vi "CSGaussmeter.setactValue.vi"(0 "VisaCluster":T7, 7 "setValues":T6 {"Set_Rel"."Numeric" format="%#_4f"; "Set_upper"."Numeric" format="%#_4f"; "Set_lower"."Numeric" format="%#_4f"}, 11 "error in":errorcluster) -> (4 "VisaCluster 2":T7, 8 "setValues":T6 {"Set_Rel"."Numeric" format="%#_4f"; "Set_upper"."Numeric" format="%#_4f"; "Set_lower"."Numeric" format="%#_4f"}, 15 "error out":errorcluster)   [LabVIEW 2014, in "CSGaussmeter.lvlib"]
uses:
  CSGaussmeter.lvlib
  CSinstr.lib/FH_55/TypeDef/VisaCluster.ctl
  CSinstr.lib/FH_55/TypeDef/Unit.ctl
  CSinstr.lib/FH_55/TypeDef/Temp_Unit.ctl
  CSinstr.lib/FH_55/TypeDef/Max.ctl
  CSinstr.lib/FH_55/TypeDef/Range.ctl
  CSinstr.lib/FH_55/TypeDef/Unit2.ctl
  CSinstr.lib/FH_55/FH 55.lvlib
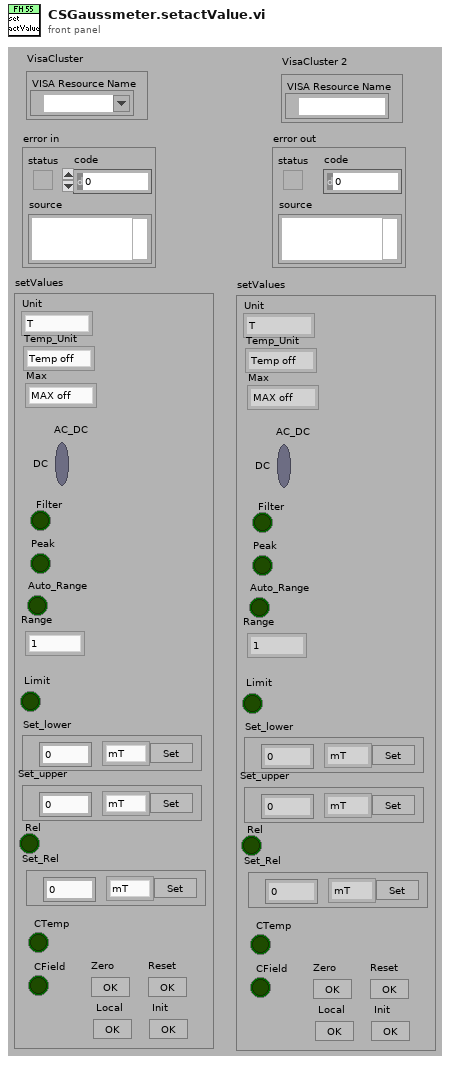
[diagram p1: front panel]
types:
  T1 = typedef "FH 55.lvlib/Unit.ctl" = enum16{"T", "G", "A/m"}
  T2 = typedef "FH 55.lvlib/Temp_Unit.ctl" = enum16{"Temp off", "Celsius", "Fahrenheit"}
  T3 = typedef "FH 55.lvlib/Max.ctl" = enum16{"MAX off", "Show MAX", "MAX/MIN"}
  T4 = typedef "FH 55.lvlib/Range.ctl" = enum16{"1", "2", "3", "4", "5", "6", "7"}
  T5 = typedef "FH 55.lvlib/Unit2.ctl" = enum16{"mT", "G", "kA/m"}
  T6 = cluster{" Limit":bool, "Unit ":T1, "Temp_Unit":T2, "Max":T3, " Filter":bool, " Peak":bool, " Auto_Range":bool, "Range":T4, " Rel":bool, " CTemp":bool, " CField":bool, "AC_DC ":bool, "Set_lower":cluster{"Numeric":dbl, "Cancel Button":bool, "Unit":T5}, "Set_upper":cluster{"Numeric":dbl, "Cancel Button":bool, "Unit":T5}, "Set_Rel":cluster{"Numeric":dbl, "Cancel Button":bool, "Unit":T5}, "Zero":bool, " Local":bool, "Reset":bool, " Init":bool}
  T7 = typedef "FH 55.lvlib/VisaCluster.ctl" = cluster{"VISA Resource Name":refnum<visa-resource-name>}
  T8 = cluster{"Numeric":dbl, "Cancel Button":bool, "Unit":T5}
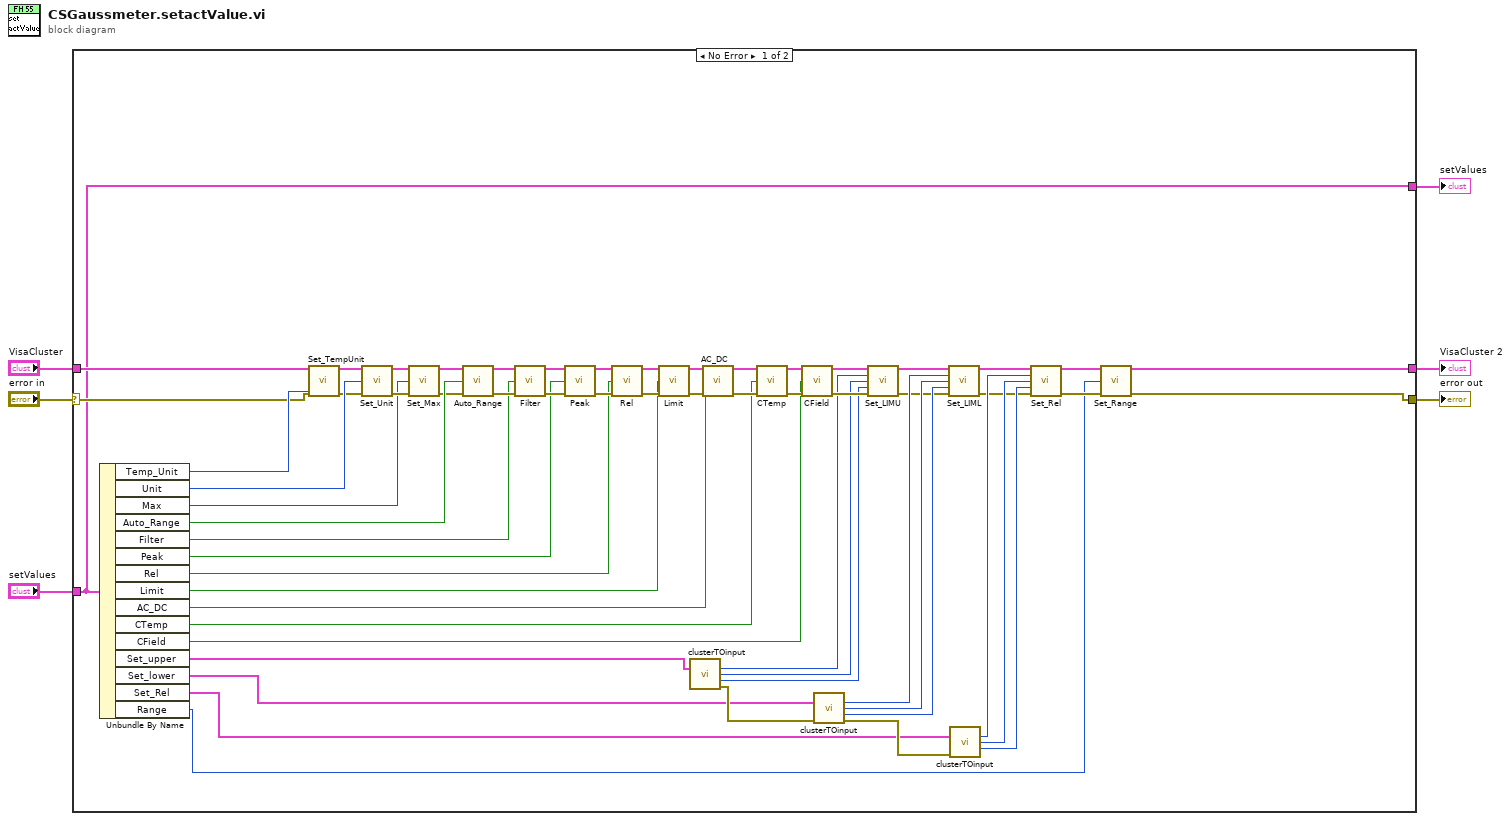
[diagram p0: block diagram]
diagram:
  n1 = case shown="No Error" "error in" {
    selector: "error in" -> [w15 w68]
    tunnel: [w13 w68] -> w5
    tunnel: "setValues" -> [w7 w66]
    tunnel: "VisaCluster" -> [w65 w67]
    tunnel: [w7 w66] -> w2
    tunnel: [w11 w67] -> w1
    frame No Error {
      n2 = Unbundle By Name(w7) -> ("Temp_Unit"=w43:T2, "Unit"=w42:T1, "Max"=w41:T3, "Auto_Range"=w40:bool, "Filter"=w39:bool, "Peak"=w38:bool, "Rel"=w37:bool, "Limit"=w36:bool, "AC_DC"=w35:bool, "CTemp"=w34:bool, "CField"=w33:bool, "Set_upper"=w32:T8, "Set_lower"=w26:T8, "Set_Rel"=w22:T8, "Range"=w10:T4)
      n3 = call "Set_TempUnit.vi"("VisaCluster"=w65, "Temp_Unit"=w43, "error in (no error)"=w15) -> ("VisaCluster"=w9:T7, "error out"=w8:errorcluster)  [unwired: 9 in, 2 out]
      n4 = call "Set_Unit.vi"("VisaCluster"=w9, "Unit"=w42, "error in (no error)"=w8) -> ("VisaCluster"=w49:T7, "error out"=w48:errorcluster)  [unwired: 9 in, 2 out]
      n5 = call "Set_Max.vi"("VisaCluster"=w49, "Max"=w41, "error in (no error)"=w48) -> ("VisaCluster"=w54:T7, "error out"=w18:errorcluster)  [unwired: 9 in, 2 out]
      n6 = call "Auto_Range.vi"("VisaCluster"=w54, "Auto_Range"=w40, "error in (no error)"=w18) -> ("VisaCluster"=w64:T7, "error out"=w59:errorcluster)  [unwired: 8 in, 3 out]
      n7 = call "Filter.vi"("VisaCluster"=w64, "Filter"=w39, "error in (no error)"=w59) -> ("VisaCluster"=w63:T7, "error out"=w58:errorcluster)  [unwired: 8 in, 3 out]
      n8 = call "Peak.vi"("VisaCluster"=w63, "Peak"=w38, "error in (no error)"=w58) -> ("VisaCluster"=w62:T7, "error out"=w57:errorcluster)  [unwired: 8 in, 3 out]
      n9 = call "Rel.vi"("VisaCluster"=w62, "Rel"=w37, "error in (no error)"=w57) -> ("VisaCluster"=w61:T7, "error out"=w56:errorcluster)  [unwired: 8 in, 3 out]
      n10 = call "Limit.vi"("VisaCluster"=w61, "Limit"=w36, "error in (no error)"=w56) -> ("VisaCluster"=w60:T7, "error out"=w55:errorcluster)  [unwired: 9 in, 2 out]
      n11 = call "clusterTOinput.vi"("Set_Rel"=w32) -> ("Range"=w31:T4, "Numeric"=w30:i32, "Unit"=w29:T1, "error out"=w28:errorcluster)  [unwired: 11 in]
      n12 = call "AC_DC.vi"("VisaCluster"=w60, "AC_DC"=w35, "error in (no error)"=w55) -> ("VisaCluster"=w53:T7, "error out"=w51:errorcluster)  [unwired: 8 in, 3 out]
      n13 = call "CTemp.vi"("VisaCluster"=w53, "CTemp"=w34, "error in (no error)"=w51) -> ("VisaCluster"=w52:T7, "error out"=w50:errorcluster)  [unwired: 9 in, 2 out]
      n14 = call "CField.vi"("VisaCluster"=w52, "CField"=w33, "error in (no error)"=w50) -> ("VisaCluster"=w46:T7, "error out"=w47:errorcluster)  [unwired: 9 in, 2 out]
      n15 = call "clusterTOinput.vi"("Set_Rel"=w26, "error in (no error)"=w28) -> ("Range"=w25:T4, "Numeric"=w24:i32, "Unit"=w23:T1, "error out"=w27:errorcluster)  [unwired: 10 in]
      n16 = call "Set_LIMU.vi"("VisaCluster"=w46, "Range"=w31, "Ziffern"=w30, "Unit"=w29, "error in (no error)"=w47) -> ("VisaCluster"=w45:T7, "error out"=w17:errorcluster)  [unwired: 8 in, 1 out]
      n17 = call "Set_LIML.vi"("VisaCluster"=w45, "Range"=w25, "Ziffern"=w24, "Unit"=w23, "error in (no error)"=w17) -> ("VisaCluster"=w44:T7, "error out"=w16:errorcluster)  [unwired: 8 in, 1 out]
      n18 = call "clusterTOinput.vi"("Set_Rel"=w22, "error in (no error)"=w27) -> ("Range"=w21:T4, "Numeric"=w20:i32, "Unit"=w19:T1)  [unwired: 10 in, 1 out]
      n19 = call "Set_Rel.vi"("VisaCluster"=w44, "Range"=w21, "Numeric"=w20, "Unit"=w19, "error in (no error)"=w16) -> ("VisaCluster"=w12:T7, "error out"=w14:errorcluster)  [unwired: 8 in, 1 out]
      n20 = call "Set_Range.vi"("VisaCluster"=w12, "Range"=w10, "error in (no error)"=w14) -> ("VisaCluster"=w11:T7, "error out"=w13:errorcluster)  [unwired: 9 in, 2 out]
    }
    frame Error {
    }
  }
  "error out" <- w5
  "VisaCluster 2" <- w1
  "setValues" <- w2
